vi "drive_simple_relative.vi"(6 "fast":bool, 7 "motor power":dbl, 8 "right distance":dbl, 9 "left distance":dbl, 10 "reinit":bool, 11 "distance target":dbl) -> (1 "right power":dbl, 2 "left power":dbl, 3 "done":bool)   [LabVIEW 2014]
panel:
  in  "rear left bias factor":dbl=0.97
  in  "forward right bias factor":dbl=0.97
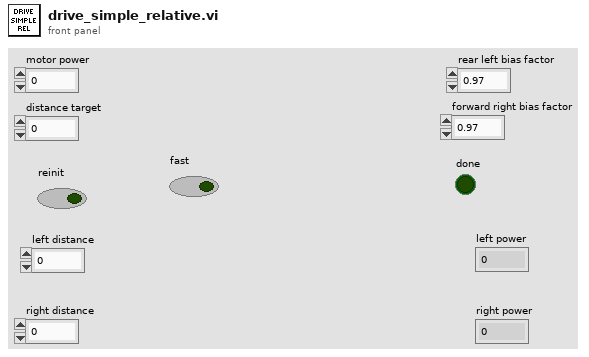
[diagram p1: front panel]
types:
  T1 = cluster{"left distance":dbl, "right distance":dbl}
  T2 = cluster{"distance target":dbl, "distance target":dbl}
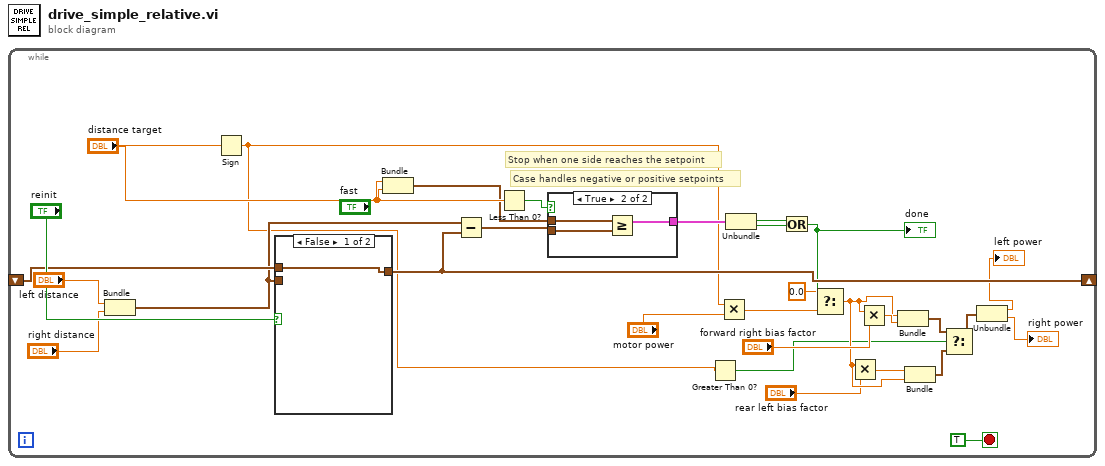
[diagram p0: block diagram]
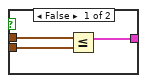
[diagram p2: hidden frame]
diagram:
  n1 = while {
    shift-right: [w23] -> _
    shift-left: _ -> [w28]
    stop <- TRUE stop-if-true
    # "Case handles negative or positive setpoints"
    # "Stop when one side reaches the setpoint"
    n2 = Bundle("left distance"="left distance", "right distance"="right distance") -> (w24:T1)  [unwired: 1 in]
    n3 = Sign(1:"distance target") -> (0:w2:dbl)
    n4 = case shown="False" "reinit" {
      tunnel: [w37 w38] -> w23
      tunnel: w24 -> [_ w38]
      tunnel: w28 -> [w37 _]
      frame False {
      }
      frame True {
      }
    }
    n5 = Bundle("distance target"="distance target", "distance target"="distance target") -> (w17:T2)  [unwired: 1 in]
    n6 = Subtract(x=w24, y=w23) -> (x-y=w16:T1)
    n7 = Less Than 0?(x="distance target") -> (x < 0?=w19:bool)
    n8 = case shown="True" w19 {
      tunnel: w17 -> [w33 w36]
      tunnel: w16 -> [w32 w35]
      tunnel: [w31 w34] -> w22
      frame False {
        n9 = Less Or Equal?(x=w33, y=w32) -> (x <= y?=w31:cluster{bool, bool})
      }
      frame True {
        n10 = Greater Or Equal?(x=w36, y=w35) -> (x >= y?=w34:cluster{bool, bool})
      }
    }
    n11 = Greater Than 0?(x=w2) -> (x > 0?=w1:bool)
    n12 = Multiply(x=w2, y="motor power") -> (x*y=w15:dbl)
    n13 = Unbundle(w22) -> (w21:bool, w20:bool)
    n14 = Or(x=w21, y=w20) -> (x .or. y?=w14:bool)
    "done" <- w14
    n15 = Select(t=0.0, s=w14, f=w15) -> (s? t:f=w10:dbl)
    n16 = Multiply(x=w10, y="rear left bias factor") -> (x*y=w9:dbl)
    n17 = Multiply(x=w10, y="forward right bias factor") -> (x*y=w11:dbl)
    n18 = Bundle("t"=w10, w11) -> (w7:cluster{"t":dbl, dbl})  [unwired: 1 in]
    n19 = Bundle(w9, "t"=w10) -> (w6:cluster{dbl, "t":dbl})  [unwired: 1 in]
    n20 = Select(t=w7, s=w1, f=w6) -> (s? t:f=w5:cluster{"t":dbl, "t":dbl})
    n21 = Unbundle(w5) -> ("t"=→"left power":dbl, "t"=→"right power":dbl)
  }
